vi "Day08-03.vi"() -> ()   [LabVIEW 2021]
uses:
  <vilib>/DAQmx/read.llb/DAQmx Read (Analog 1D Wfm NChan NSamp).vi
  <vilib>/DAQmx/miscellaneous.llb/DAQmx Fill In Error Info.vi
panel:
  out "data":waveform(dbl)[](graph) caption="데이터"
  in  "stop":bool caption="정지"
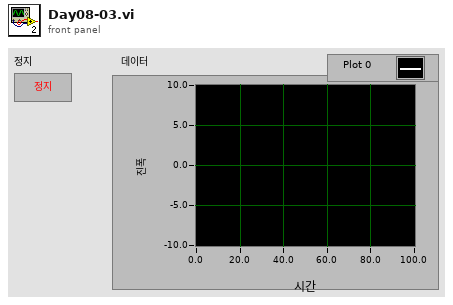
[diagram p1: front panel]
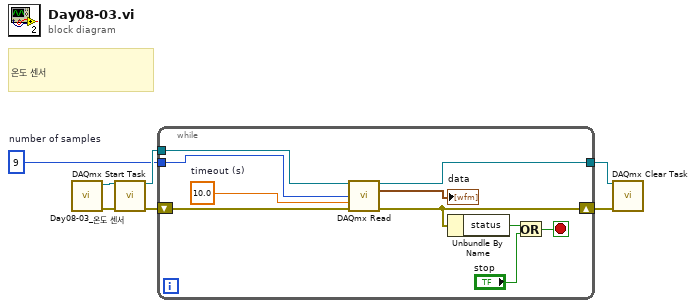
[diagram p0: block diagram]
diagram:
  w5 = 9  # number of samples
  # "온도 센서"
  n1 = call "Day08-03_온도 센서.vi"() -> ("error out"=w1:errorcluster, "task out"=w2:refnum<k21>)  [unwired: 10 in]
  n2 = call <vilib>:"DAQmx Start Task.vi"("task/channels in"=w2, "error in"=w1) -> ("task out"=w7:refnum<k21>, "error out"=w6:errorcluster)  [unwired: 12 in]
  n3 = while "While 루프" {
    tunnel: w7 -> [w17]
    tunnel: w5 -> [w13]
    tunnel: [w14] -> w3
    shift-right: [w11] -> w4
    shift-left: w6 -> [w16]
    stop <- w10 stop-if-true
    w8 = 10.0  # timeout (s)
    n4 = call-poly <vilib>:"DAQmx Read.vi"("task/channels in"=w17, "number of samples per channel"=w13, "timeout"=w8, "error in"=w16) -> ("task out"=w14:refnum<k21>, "data"=→"data":waveform(dbl)[], "error out"=w11:errorcluster)  [unwired: 9 in]
    n5 = Unbundle By Name(w11) -> ("status"=w12:bool)
    n6 = Or(x=w12, y="stop") -> (x .or. y?=w10:bool)
  }
  n7 = call <vilib>:"DAQmx Clear Task.vi"("task in"=w3, "error in"=w4) -> ()  [unwired: 13 in, 1 out]
